vi "Build Excel File.vi"(6 "close report? (T)":bool=TRUE, 7 "Gas":bool, 8 "error in":errorcluster, 9 "Language":T2, 10 "Raw data":string[][](table), 11 "Information":T1) -> (0 "error out":errorcluster, 1 "Excel path":path, 2 "PDF path out":path)   [LabVIEW 2016]
uses:
  Controls/Language Control.ctl
  Controls/Information_tab_type.ctl
  Controls/ctrlReportStates.ctl
  Controls/ctrlReportData.ctl
  <vilib>/Utility/NIReport.llb/NI_report.lvclass
  <vilib>/Utility/NIReport.llb/Excel/NI_Excel.lvclass
  <vilib>/addons/_office/NI_ReportGenerationToolkit.lvlib
  <vilib>/Utility/sysdir.llb/System Directory Type.ctl
panel:
  out "Pass?":bool
  out "rows":i32[](array[numeric])
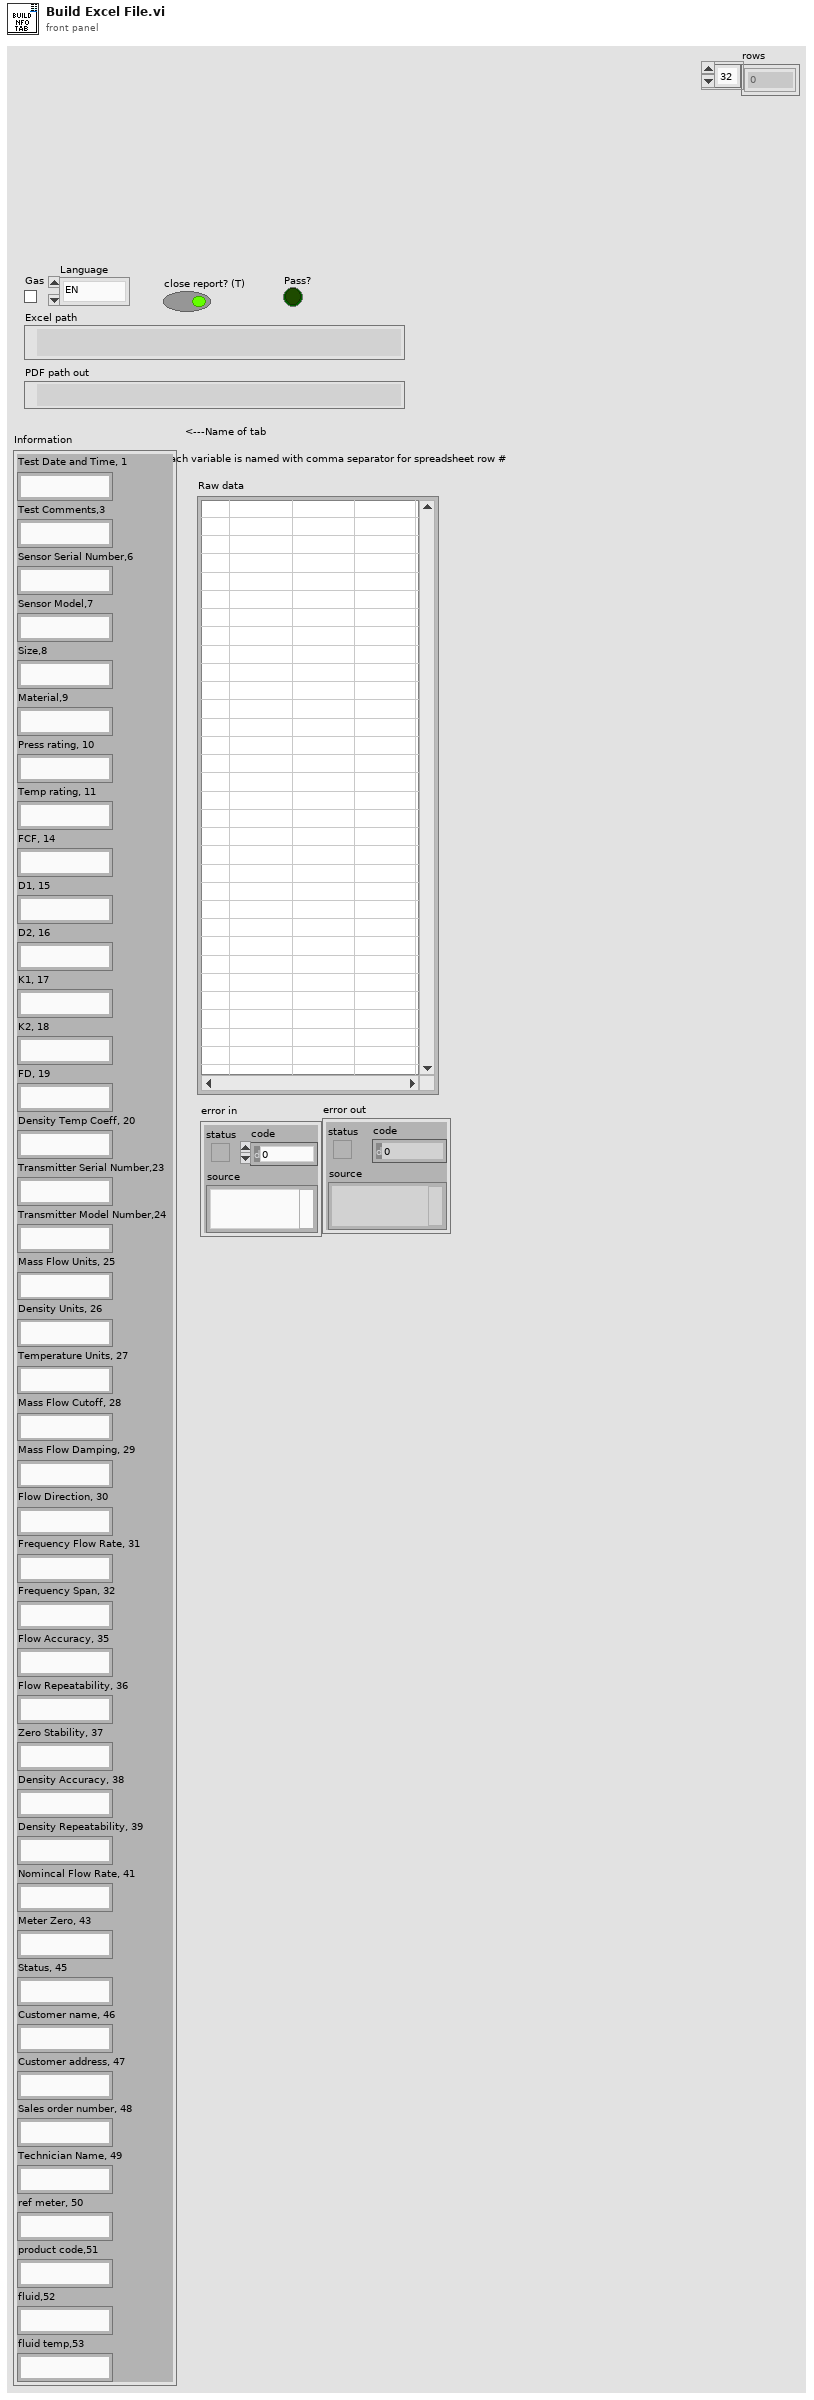
[diagram p1: front panel]
types:
  T1 = typedef "Information_tab_type.ctl" = cluster{"Test Date and Time, 1":string, "Test Comments,3":string, "Sensor Serial Number,6":string, "Sensor Model,7":string, "Size,8":string, "Material,9":string, "Press rating, 10":string, "Temp rating, 11":string, "FCF, 14":string, "D1, 15":string, "D2, 16":string, "K1, 17":string, "K2, 18":string, "FD, 19":string, "Density Temp Coeff, 20":string, "Transmitter Serial Number,23":string, "Transmitter Model Number,24":string, "Mass Flow Units, 25":string, "Density Units, 26":string, "Temperature Units, 27":string, "Mass Flow Cutoff, 28":string, "Mass Flow Damping, 29":string, "Flow Direction, 30":string, "Frequency Flow Rate, 31":string, "Frequency Span, 32":string, "Flow Accuracy, 35":string, "Flow Repeatability, 36":string, "Zero Stability, 37":string, "Density Accuracy, 38":string, "Density Repeatability, 39":string, "Nomincal Flow Rate, 41":string, "Meter Zero, 43":string, "Status, 45":string, "Customer name, 46":string, "Customer address, 47":string, "Sales order number, 48":string, "Technician Name, 49":string, "ref meter, 50":string, "product code,51":string, "fluid,52":string, "fluid temp,53":string}
  T2 = typedef "Language Control.ctl" = enum16{"EN", "ES", "FR", "RU"}
  T3 = typedef "ctrlReportData.ctl" = cluster{"ReportTemplatePath":path, "ReportFolderPath":path, "Information":T1, "Raw data":string[][], "ReportRef":refnum<class "NI_report.lvclass">, "Pass?":bool}
  T4 = typedef "ctrlReportStates.ctl" = enum16{"GetTemplatePath", "GetInputControls", "NewReport", "Update-SSCStyle", "Update-Information", "Update-RawData", "ExportReport", "DisposeReport"}
  T5 = cluster{"Current Path":path, "DataFiles Path":path, "ReportFiles Path":path, "SupportFiles Path":path, "ReportTemplate Path":path, "Sample_pulses_VIT_Path":path, "Sample_current_VIT_Path":path, "Sample_MODBUS_VIT_Path":path}
  T6 = enum16{"maximized", "minimized", "normal", "no change"}
  T7 = enum16{"Standard Report", "HTML", "Word", "Excel"}
  T8 = typedef "System Directory Type.ctl" = i32
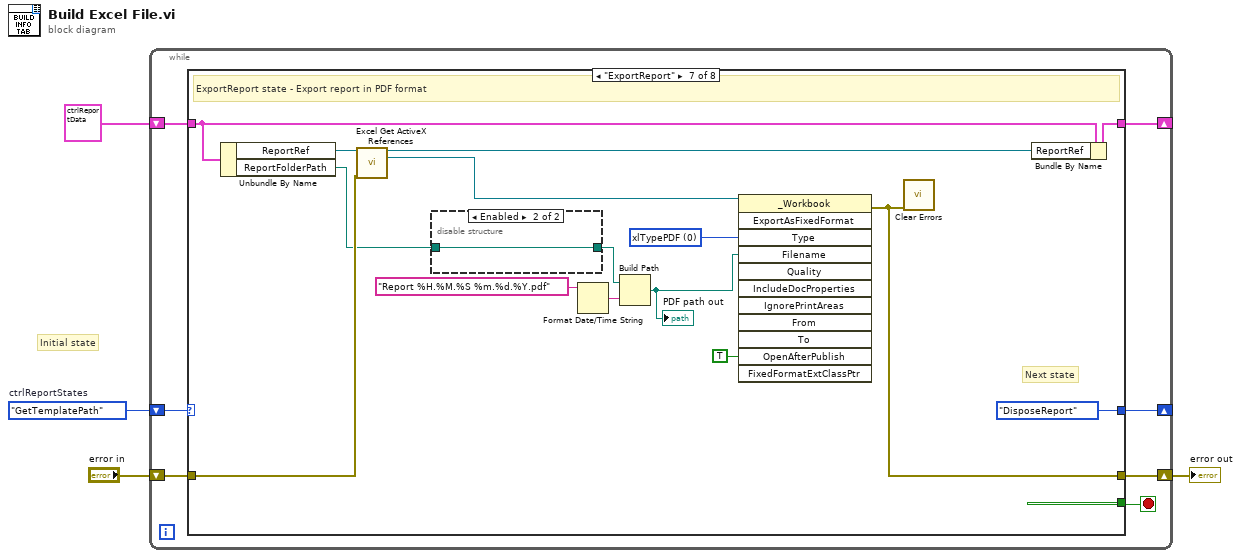
[diagram p0: block diagram]
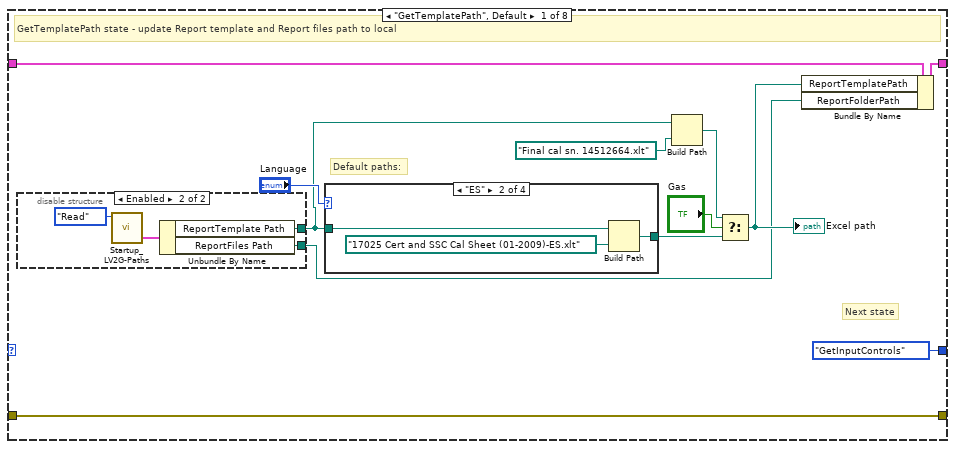
[diagram p2: hidden frame]
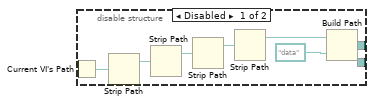
[diagram p3: hidden frame]
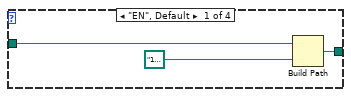
[diagram p4: hidden frame]
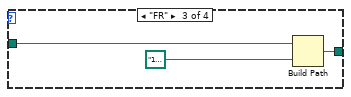
[diagram p5: hidden frame]
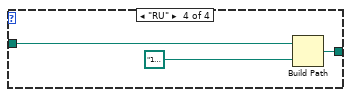
[diagram p6: hidden frame]
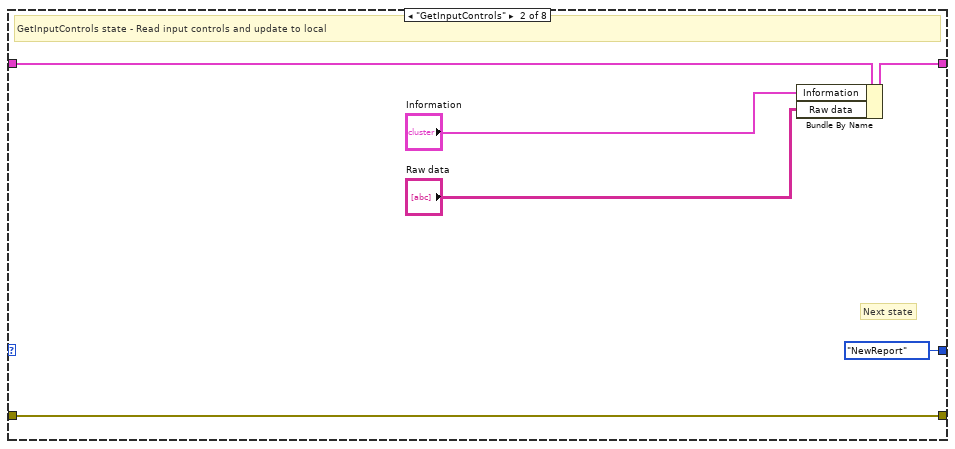
[diagram p7: hidden frame]
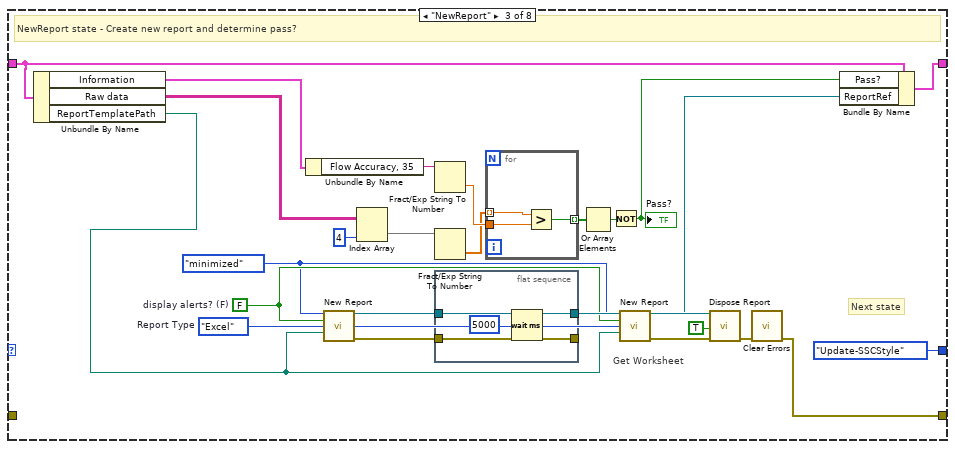
[diagram p8: hidden frame]
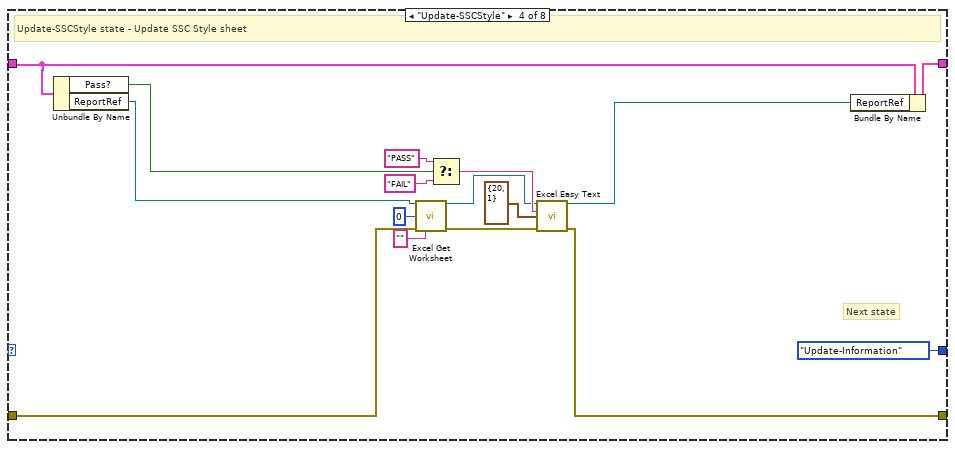
[diagram p9: hidden frame]
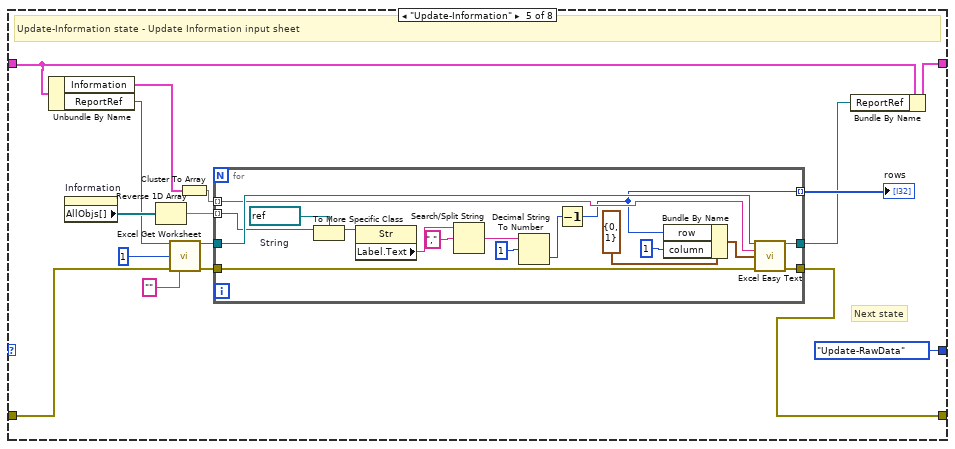
[diagram p10: hidden frame]
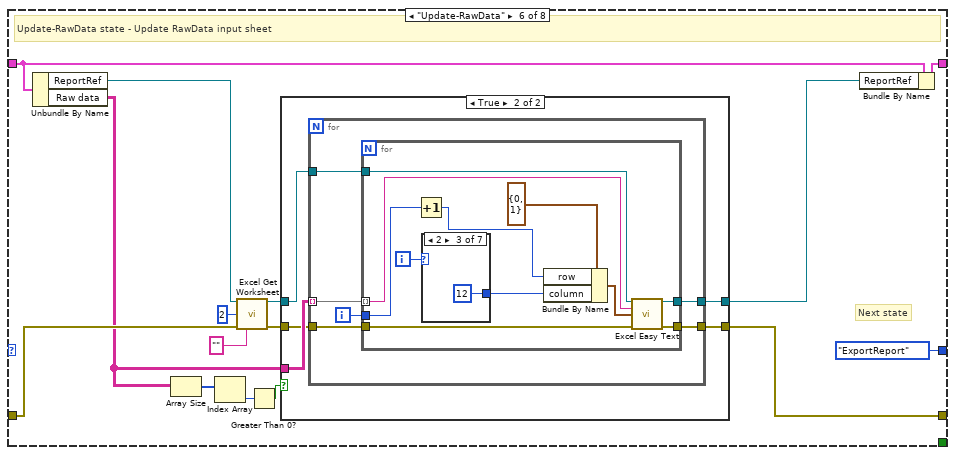
[diagram p11: hidden frame]
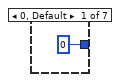
[diagram p13: hidden frame]
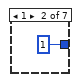
[diagram p14: hidden frame]
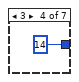
[diagram p15: hidden frame]
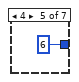
[diagram p16: hidden frame]
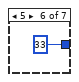
[diagram p17: hidden frame]
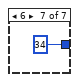
[diagram p18: hidden frame]
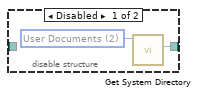
[diagram p19: hidden frame]
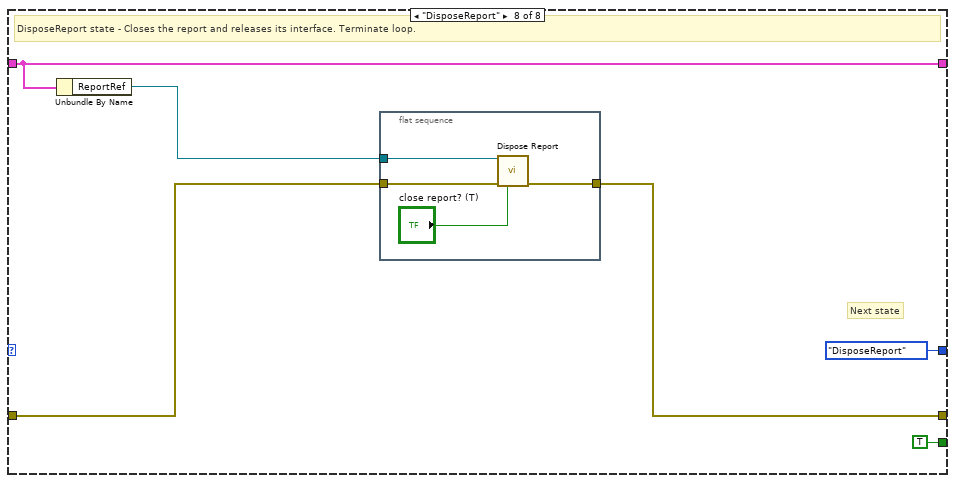
[diagram p20: hidden frame]
diagram:
  w4 = ctrlReportStates."GetTemplatePath"  # ctrlReportStates
  # "Initial state"
  n1 = while {
    shift-right: [w10] -> _
    shift-left: w4 -> [w11]
    shift-right: [w7] -> _
    shift-left: T3 {"ReportTemplatePath"=path "", "ReportFolderPath"=path "", "Information"={"Test Date and Time, 1"="", "Test Comments,3"="", "Sensor Serial Number,6"="", "Sensor Model,7"="", "Size,8"="", "Material,9"="", "Press rating, 10"="", "Temp rating, 11"="", "FCF, 14"="", "D1, 15"="", "D2, 16"="", "K1, 17"="", "K2, 18"="", "FD, 19"="", "Density Temp Coeff, 20"="", "Transmitter Serial Number,23"="", "Transmitter Model Number,24"="", "Mass Flow Units, 25"="", "Density Units, 26"="", "Temperature Units, 27"="", "Mass Flow Cutoff, 28"="", "Mass Flow Damping, 29"="", "Flow Direction, 30"="", "Frequency Flow Rate, 31"="", "Frequency Span, 32"="", "Flow Accuracy, 35"="", "Flow Repeatability, 36"="", "Zero Stability, 37"="", "Density Accuracy, 38"="", "Density Repeatability, 39"="", "Nomincal Flow Rate, 41"="", "Meter Zero, 43"="", "Status, 45"="", "Customer name, 46"="", "Customer address, 47"="", "Sales order number, 48"="", "Technician Name, 49"="", "ref meter, 50"="", "product code,51"="", "fluid,52"="", "fluid temp,53"=""}, "Raw data"=[], "ReportRef"=refnum, "Pass?"=FALSE} ("ctrlReportData") -> [w8]
    shift-right: [w6] -> w1
    shift-left: "error in" -> [w5]
    stop <- w9 stop-if-true
    n2 = case shown="\"ExportReport\"" w11 {
      tunnel: [ctrlReportStates."GetInputControls" ("ctrlReportStates") ctrlReportStates."NewReport" ("ctrlReportStates") ctrlReportStates."Update-SSCStyle" ("ctrlReportStates") ctrlReportStates."Update-Information" ("ctrlReportStates") ctrlReportStates."Update-RawData" ("ctrlReportStates") ctrlReportStates."ExportReport" ("ctrlReportStates") ctrlReportStates."DisposeReport" ("ctrlReportStates") ctrlReportStates."DisposeReport" ("ctrlReportStates")] -> w10
      tunnel: [_ _ _ _ _ _ _ TRUE] -> w9
      tunnel: w8 -> [w20 w51 w59 w99 w115 w140 w192 w200]
      tunnel: [w19 w50 w77 w98 w114 w139 w191 w200] -> w7
      tunnel: [w15 w47 w53 w84 w101 w134 w181 w197] -> w6
      tunnel: w5 -> [w15 w47 _ w85 w102 w137 w182 w198]
      frame "GetTemplatePath", Default {
        # "Next state"
        # "Default paths:"
        # "GetTemplatePath state - update Report template and Report files path to local"
        n3 = disable-structure shown="Enabled" {
          disable-tunnel: [w30 w32] -> w13
          disable-tunnel: [_ w31] -> w16
          frame Disabled {
            n4 = Current VI's Path() -> (path=w28:path)
            n5 = Strip Path(path=w28) -> (stripped path=w27:path)  [unwired: 1 out]
            n6 = Strip Path(path=w27) -> (stripped path=w26:path)  [unwired: 1 out]
            n7 = Strip Path(path=w26) -> (stripped path=w25:path)  [unwired: 1 out]
            n8 = Strip Path(path=w25) -> (stripped path=w24:path)  [unwired: 1 out]
            n9 = Build Path(base path=w24, name or relative path=path "data") -> (appended path=w30:path)
          }
          frame Enabled {
            n10 = call "Startup_LV2G-Paths.vi"("Action"=enum16{"Read", "Write"}."Read") -> ("Paths"=w34:T5)  [unwired: 9 in, 1 out]
            n11 = Unbundle By Name(w34) -> ("ReportTemplate Path"=w32:path, "ReportFiles Path"=w31:path)
          }
        }
        n12 = case shown="\"ES\"" "Language" {
          tunnel: [w37 w40 w43 w46] -> w22
          tunnel: w13 -> [w35 w39 w42 w45]
          frame "EN", Default {
            n13 = Build Path(base path=w35, name or relative path=path "17025 Cert and SSC Cal Sheet (01-2009)-EN.xlt") -> (appended path=w37:path)
          }
          frame "ES" {
            n14 = Build Path(base path=w39, name or relative path=path "17025 Cert and SSC Cal Sheet (01-2009)-ES.xlt") -> (appended path=w40:path)
          }
          frame "FR" {
            n15 = Build Path(base path=w42, name or relative path=path "17025 Cert and SSC Cal Sheet (01-2009)-FR.xlt") -> (appended path=w43:path)
          }
          frame "RU" {
            n16 = Build Path(base path=w45, name or relative path=path "17025 Cert and SSC Cal Sheet (01-2009)-RU.xlt") -> (appended path=w46:path)
          }
        }
        n17 = Build Path(base path=w13, name or relative path=path "Final cal sn. 14512664.xlt") -> (appended path=w12:path)
        n18 = Select(t=w12, s="Gas", f=w22) -> (s? t:f=w18:path)
        "Excel path" <- w18
        n19 = Bundle By Name(cluster=w20, "ReportTemplatePath"=w18, "ReportFolderPath"=w16) -> (w19:T3)
      }
      frame "GetInputControls" {
        # "Next state"
        # "GetInputControls state - Read input controls and update to local"
        n20 = Bundle By Name(cluster=w51, "Information"="Information", "Raw data"="Raw data") -> (w50:T3)
      }
      frame "NewReport" {
        w70 = FALSE  # display alerts? (F)
        w69 = T6."minimized" ("window state (normal)")
        w71 = T7."Excel"  # Report Type
        # "Next state"
        # "Get Worksheet"
        # "NewReport state - Create new report and determine pass?"
        n21 = Unbundle By Name(w59) -> ("Information"=w56:T1, "Raw data"=w55:string[][], "ReportTemplatePath"=w54:path)
        n22 = Unbundle By Name(w56) -> ("Flow Accuracy, 35"=w63:string)
        n23 = call <vilib>:"New Report.vi"("window state (normal)"=w69, "display alerts? (F)"=w70, "report type"=w71, "template (empty)"=w54) -> ("report out"=w72:refnum<class "NI_report.lvclass">, "error out"=w73:errorcluster)  [unwired: 10 in]
        n24 = Index Array(array=w55, index (col)=4 ("disabled index (col)")) -> (element=w61:string[])  [unwired: 1 in]
        n25 = Fract/Exp String To Number(string=w63) -> (number=w64:dbl)  [unwired: 3 in, 1 out]
        n26 = Fract/Exp String To Number(string=w61) -> (number=w62:dbl[])  [unwired: 3 in, 1 out]
        n27 = flat-sequence {
          tunnel: w72 -> [w80]
          tunnel: w73 -> [w79]
          tunnel: [w80] -> w74
          tunnel: [w79] -> _
          frame #0 {
            n28 = Wait (ms)(milliseconds to wait=u32 5000) -> ()  [unwired: 1 out]
          }
        }
        n29 = for {
          tunnel: w62 -> [w83] mode=indexing
          tunnel: w64 -> [w82]
          tunnel: [w81] -> w65 mode=indexing
          n30 = Greater?(x=w83, y=w82) -> (0:w81:bool)
        }
        n31 = Or Array Elements(Boolean array=w65) -> (logical OR=w66:bool)
        n32 = Not(x=w66) -> (.not. x?=w58:bool)
        "Pass?" <- w58
        n33 = call <vilib>:"New Report.vi"("window state (normal)"=w69, "display alerts? (F)"=w70, "report type"=w71, "template (empty)"=w54) -> ("report out"=w57:refnum<class "NI_report.lvclass">, "error out"=w75:errorcluster)  [unwired: 10 in]
        n34 = call-dynamic "Dispose Report.vi"("report in"=w74, "error in (no error)"=w75, "close report? (T)"=TRUE) -> ("error out"=w68:errorcluster)  [unwired: 12 in]
        n35 = call <vilib>:"Clear Errors.vi"("error in (no error)"=w68) -> ("error out"=w53:errorcluster)  [unwired: 5 in, 1 out]
        n36 = Bundle By Name(cluster=w59, "Pass?"=w58, "ReportRef"=w57) -> (w77:T3)
      }
      frame "Update-SSCStyle" {
        # "Next state"
        # "Update-SSCStyle state - Update SSC Style sheet"
        n37 = Unbundle By Name(w99) -> ("Pass?"=w88:bool, "ReportRef"=w89:refnum<class "NI_report.lvclass">)
        n38 = call <vilib>:"Excel Get Worksheet.vi"("report in"=w89, "worksheet index (0)"=0, "error in (no error)"=w85, "name (\"\")"="" ("name (\"\")")) -> ("report out"=w94:refnum<class "NI_report.lvclass">, "error out"=w97:errorcluster)  [unwired: 10 in]
        n39 = Select(t="PASS", s=w88, f="FAIL") -> (s? t:f=w95:string)
        n40 = call <vilib>:"Excel Easy Text.vi"("report in"=w94, "text"=w95, "start (-1, -1)"=cluster{"row":i32, "column":i32} {"row"=20, "column"=1}, "error in (no error)"=w97) -> ("report out"=w87:refnum<class "NI_report.lvclass">, "error out"=w84:errorcluster)  [unwired: 7 in, 3 out]
        n41 = Bundle By Name(cluster=w99, "ReportRef"=w87) -> (w98:T3)
      }
      frame "Update-Information" {
        # "Next state"
        # "Update-Information state - Update Information input sheet"
        n42 = Unbundle By Name(w115) -> ("Information"=w104:T1, "ReportRef"=w103:refnum<class "NI_report.lvclass">)
        n43 = property on="Information" class="Clust (strict)"() -> ("AllObjs[]"=w110:refnum<vi>[])  [unwired: 2 in, 2 out]
        n44 = Reverse 1D Array(array=w110) -> (reversed array=w111:refnum<vi>[])
        n45 = call <vilib>:"Excel Get Worksheet.vi"("report in"=w103, "worksheet index (0)"=1, "error in (no error)"=w102, "name (\"\")"="" ("name (\"\")")) -> ("report out"=w106:refnum<class "NI_report.lvclass">, "error out"=w105:errorcluster)  [unwired: 10 in]
        n46 = Cluster To Array(cluster=w104) -> (array=w109:string[])
        n47 = for {
          tunnel: w106 -> [w132]
          tunnel: w105 -> [w131]
          tunnel: [w130] -> w101
          tunnel: [w129] -> w100
          tunnel: w109 -> [w128] mode=indexing
          tunnel: w111 -> [w118] mode=indexing
          tunnel: [w116] -> w112 mode=indexing
          w127 = refnum<vi> refnum  # String
          n48 = To More Specific Class(target class=w127, reference=w118) -> (specific class reference=w126:refnum<vi>)  [unwired: 1 in, 1 out]
          n49 = property class="Str"(reference=w126) -> ("Label.Text"=w125:string)  [unwired: 1 in, 2 out]
          n50 = Search/Split String(string=w125, search string/char (-)=",") -> (match + rest of string=w123:string)  [unwired: 1 in, 2 out]
          n51 = Decimal String To Number(string=w123, offset=1) -> (number=w121:i32)  [unwired: 1 in, 1 out]
          n52 = Decrement(x=w121) -> (x-1=w116:i32)
          n53 = Bundle By Name(cluster=cluster{"row":i32, "column":i32} {"row"=0, "column"=1} ("start (-1, -1)"), "row"=w116, "column"=1) -> (w119:cluster{"row":i32, "column":i32})
          n54 = call <vilib>:"Excel Easy Text.vi"("report in"=w132, "text"=w128, "start (-1, -1)"=w119, "error in (no error)"=w131) -> ("report out"=w129:refnum<class "NI_report.lvclass">, "error out"=w130:errorcluster)  [unwired: 7 in, 3 out]
        }
        "rows" <- w112
        n55 = Bundle By Name(cluster=w115, "ReportRef"=w100) -> (w114:T3)
      }
      frame "Update-RawData" {
        # "Next state"
        # "Update-RawData state - Update RawData input sheet"
        n56 = Unbundle By Name(w140) -> ("ReportRef"=w138:refnum<class "NI_report.lvclass">, "Raw data"=w136:string[][])
        n57 = Array Size(array=w136) -> (size(s)=w145:i32[])
        n58 = Index Array(array=w145) -> (element=w147:i32)  [unwired: 1 in]
        n59 = call <vilib>:"Excel Get Worksheet.vi"("report in"=w138, "worksheet index (0)"=2, "error in (no error)"=w137, "name (\"\")"="" ("name (\"\")")) -> ("report out"=w143:refnum<class "NI_report.lvclass">, "error out"=w144:errorcluster)  [unwired: 10 in]
        n60 = Greater Than 0?(x=w147) -> (x > 0?=w146:bool)
        n61 = case shown="True" w146 {
          tunnel: w136 -> [_ w154]
          tunnel: w143 -> [w149 w153]
          tunnel: w144 -> [w148 w152]
          tunnel: [w149 w151] -> w133
          tunnel: [w148 w150] -> w134
          frame False {
          }
          frame True {
            n62 = for {
              tunnel: w154 -> [w159] mode=indexing
              tunnel: w153 -> [w158]
              tunnel: [w157] -> w151
              tunnel: w152 -> [w156]
              tunnel: [w155] -> w150
              i -> [w160]
              n63 = for {
                tunnel: w160 -> [w169]
                tunnel: w159 -> [w166] mode=indexing
                tunnel: w158 -> [w164]
                tunnel: [w163] -> w157
                tunnel: w156 -> [w162]
                tunnel: [w161] -> w155
                i -> [w167]
                n64 = Increment(x=w169) -> (x+1=w168:i32)
                n65 = case shown="2" w167 {
                  tunnel: [0 ("column") 1 ("column") 12 ("column") 14 ("column") 6 ("column") 33 ("column") 34 ("column")] -> w165
                  frame 0, Default {
                  }
                  frame 1 {
                  }
                  frame 2 {
                  }
                  frame 3 {
                  }
                  frame 4 {
                  }
                  frame 5 {
                  }
                  frame 6 {
                  }
                }
                n66 = Bundle By Name(cluster=cluster{"row":i32, "column":i32} {"row"=0, "column"=1} ("start (-1, -1)"), "row"=w168, "column"=w165) -> (w170:cluster{"row":i32, "column":i32})
                n67 = call <vilib>:"Excel Easy Text.vi"("report in"=w164, "text"=w166, "start (-1, -1)"=w170, "error in (no error)"=w162) -> ("report out"=w163:refnum<class "NI_report.lvclass">, "error out"=w161:errorcluster)  [unwired: 7 in, 3 out]
              }
            }
          }
        }
        n68 = Bundle By Name(cluster=w140, "ReportRef"=w133) -> (w139:T3)
      }
      frame "ExportReport" {
        w187 = 0 items=["xlTypePDF", "xlTypeXPS"] ("Type")
        # "Next state"
        # "ExportReport state - Export report in PDF format"
        n69 = Unbundle By Name(w192) -> ("ReportRef"=w183:refnum<class "NI_report.lvclass">, "ReportFolderPath"=w179:path)
        n70 = call <vilib>:"Excel Get ActiveX References.vi"("report in"=w183, "error in (no error)"=w182) -> ("report out"=w180:refnum<class "NI_report.lvclass">, "Excel._Workbook"=w189:refnum<k7>)  [unwired: 7 in, 5 out]
        n71 = disable-structure shown="Enabled" {
          disable-tunnel: [w195 w196] -> w190
          disable-tunnel: w179 -> [_ w196]
          frame Disabled {
            w194 = T8 2 items=["User Home"=0, "User Desktop"=1, "User Documents"=2, "User Application Data"=3, "User Preferences"=4, "User Temporary"=5, "Public Documents"=6, "Public Application Data"=7, "Public Preferences"=8, "Public Cache"=13, "System Core Libraries"=9, "System Installed Libraries"=10, "Application Files"=11, "Boot Volume Root"=12] ("system directory type")
            n72 = call <vilib>:"Get System Directory.vi"("system directory type"=w194) -> ("system directory"=w195:path)  [unwired: 10 in]
          }
          frame Enabled {
          }
        }
        n73 = Format Date/Time String(time format string (%c)="Report %H.%M.%S %m.%d.%Y.pdf") -> (date/time string=w185:string)  [unwired: 2 in]
        n74 = Build Path(base path=w190, name or relative path=w185) -> (appended path=w186:path)
        "PDF path out" <- w186
        n75 = invoke class="_Workbook" method="ExportAsFixedFormat"(reference=w189, "Type"=w187, "Filename"=w186, "OpenAfterPublish"=TRUE) -> (error out=w181:errorcluster)  [unwired: 8 in, 11 out]
        n76 = call <vilib>:"Clear Errors.vi"("error in (no error)"=w181) -> ()  [unwired: 5 in, 2 out]
        n77 = Bundle By Name(cluster=w192, "ReportRef"=w180) -> (w191:T3)
      }
      frame "DisposeReport" {
        # "Next state"
        # "DisposeReport state - Closes the report and releases its interface. Terminate loop."
        n78 = Unbundle By Name(w200) -> ("ReportRef"=w199:refnum<class "NI_report.lvclass">)
        n79 = flat-sequence {
          tunnel: w199 -> [w205]
          tunnel: w198 -> [w204]
          tunnel: [w203] -> w197
          frame #0 {
            n80 = call-dynamic "Dispose Report.vi"("report in"=w205, "error in (no error)"=w204, "close report? (T)"="close report? (T)") -> ("error out"=w203:errorcluster)  [unwired: 12 in]
          }
        }
      }
    }
  }
  "error out" <- w1
